vi "Dashboard Main.vi"() -> ()   [LabVIEW 2020]
uses:
  <vilib>/Utility/miscctls.llb/LVRowAndColumnTypeDef.ctl
  <vilib>/event_ctls.llb/eventvkey.ctl
  <vilib>/Rock Robotics/Network Tables/NT Read Numeric Array.vi
  <vilib>/Rock Robotics/Network Tables/NT Read Boolean.vi
  <vilib>/Rock Robotics/WPI/Dashboard/WPI_DashboardLogging Global.vi
panel:
  in  "Camera Settings Right":T1={"Frame Rate"=30, "Compression"=30, "Size"=1, "DB Camera Config"=FALSE} {"Frame Rate" scale=1.0..30.0; "Compression" scale=100.0..-1.0; "Size" items=["640x480", "320x240", "160x120"]}
  in  "Camera Name Right":string(combo)="No Camera Selection"
  out "Camera Perf":string
  in  "Camera Settings":T1={"Frame Rate"=30, "Compression"=30, "Size"=1, "DB Camera Config"=FALSE} {"Frame Rate" scale=1.0..30.0; "Compression" scale=100.0..-1.0; "Size" items=["640x480", "320x240", "160x120"]}
  in  "TCP":refnum<k5>
  in  "Rec Mode":enum32{"Stop", "Record", "Playback"}(radio)
  out "Robot IP":string
  out "Image Message":string="Timeout in Camera Communications"
  in  "Dashboard Tab":T2(tab)
  in  "Select Auto":string(combo)="Select Autonomous ..."
  out "NT Connection":bool
  out "MotorChart R":cluster{"Numeric":dbl, "Numeric":dbl}(graph)
  out "MotorChart L":cluster{"Numeric":dbl, "Numeric":dbl}(graph)
  out "MotorSliders R":cluster{"MotorSlide1":dbl, "MotorSlide2":dbl} {"MotorSlide2" scale=-1.0..1.0 scale format="%#_2e"; "MotorSlide1" scale=-1.0..1.0 scale format="%#_2e"}
  out "MotorSliders L":cluster{"MotorSlide1":dbl, "MotorSlide2":dbl} {"MotorSlide2" scale=-1.0..1.0 scale format="%#_2e"; "MotorSlide1" scale=-1.0..1.0 scale format="%#_2e"}
  out "Gyro":dbl(knob) scale=0.0..360.0
  out "JS1 Z":dbl(slide) scale=-1.0..1.0 scale format="%#_2e"
  out "JS1 Graph":cluster{"X":dbl, "Y":dbl}[](graph)
  out "JS1 Buttons":T3
  out "JS2 Z":dbl(slide) scale=-1.0..1.0 scale format="%#_2e"
  out "JS2 Graph":cluster{"X":dbl, "Y":dbl}[](graph)
  out "JS2 Buttons":T3
  out "Mode":T4(ring)=enum."Auto Disabled"
  out "Right Camera Perf":cluster{"Bandwidth (Mbps)":dbl, "FPS":dbl}
  out "Camera Image Right":T5(plugin-control)
  in  "DB/String 9":string
  in  "DB/String 8":string
  in  "DB/String 7":string
  in  "DB/String 6":string
  in  "DB/String 5":string
  in  "DB/String 4":string
  in  "DB/String 3":string
  in  "DB/String 2":string
  in  "DB/String 1":string
  in  "DB/String 0":string
  in  "DB/Slider 0":dbl(slide) scale=0.0..5.0
  in  "DB/Slider 1":dbl(slide) scale=0.0..5.0
  in  "DB/Slider 2":dbl(slide) scale=0.0..5.0
  in  "DB/Slider 3":dbl(slide) scale=0.0..5.0
  out "DB/LED 3":bool
  out "DB/LED 2":bool
  out "DB/LED 1":bool
  out "DB/LED 0":bool
  in  "DB/Button 3":bool
  in  "DB/Button 2":bool
  in  "DB/Button 1":bool
  in  "DB/Button 0":bool caption="New Name"
  out "Intake on?":bool
  out "Intake Sensor":bool
  out "Elevate Sensor":bool
  in  "Select Climb":string(combo)="Select Autonomous ..."
  in  "Alliance":bool
  in  "Bottom":u32(colorbox)
  out "Last":u32(colorbox)
  out "Intake % Voltage":dbl
  out "Shooter % Voltage":dbl
  in  "Shoot Equation C Value":dbl=3100.0
  in  "Test Slider":dbl(slide) scale=0.0..100.0 scale format="%#_3g"
  in  "On/Off":bool caption="Solenoid"
  in  "Test Name":u16(ring) items=["Select the test to run..."]
  in  "Test Tree":string(tree)
  in  "Motor":cluster{"Value":dbl, "Enable":bool} {"Value" scale=-1.0..1.0 scale format="%#_3g"}
  out "Progress":T6 {"Test Progress" scale=0.0..100.0}
  in  "Rev/Fwd":cluster{"Forward":bool, "Reverse":bool}
  in  "Test Ring":u16(ring) items=["Monochrome", "Color"]
  out "Cmd Status":string
  in  "Execute Command":bool
  in  "Command Params":string[][](table)
  in  "Command Selection":i32(listbox)
  in  "CheckList":i32(listbox)
  out "Tree":string(tree)
  out "Camera Image":T5(plugin-control)
  out "Background":bool
  in  "Camera Name":string(combo)="No Camera Selection"
  # "HW"
  # "HW"
  # "Joysticks"
  # "Drive Motors"
  # "Front"
  # "Right"
  # "Left"
  # "Back"
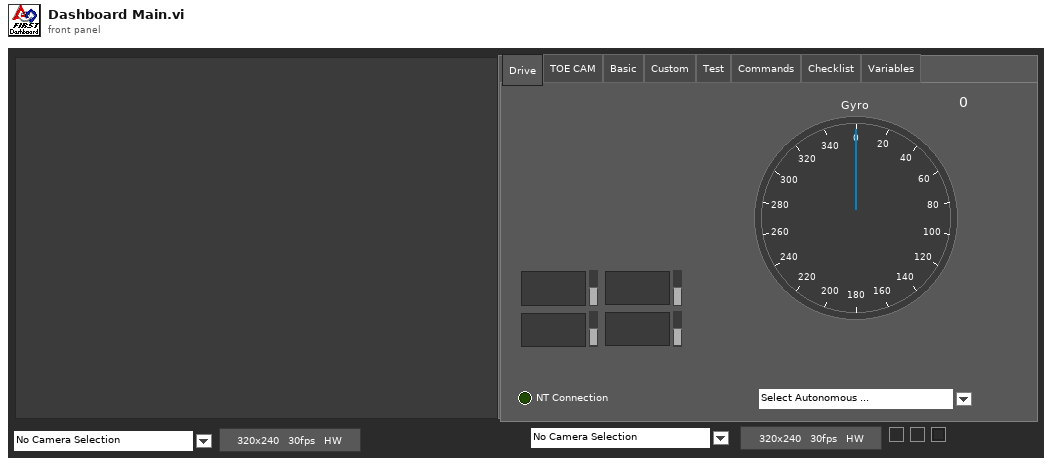
[diagram p1: front panel]
types:
  T1 = cluster{"Frame Rate":i32, "Compression":i32, "Size":u16, "DB Camera Config":bool}
  T2 = enum32{"Drive", "TOE CAM", "Basic", "Custom", "Test", "Commands", "Checklist", "Variables"}
  T3 = cluster{bool, bool, bool, bool, bool, bool, bool, bool, bool, bool, bool, bool}
  T4 = enum8{"Tele-Op Disabled", "Tele-Op Enabled", "Auto Disabled", "Auto Enabled", "Test Disabled", "Test Enabled", "Disconnected", "No Code", "E-Stop"}
  T5 = typedef "IMAQ Image.ctl" = refnum<image>
  T6 = cluster{"Test Progress":u8, "Test Progress Text":string}
  T7 = cluster{"Save Path":path, "Interval (s)":dbl, "Keep":i32}
  T8 = enum32{"Drive", "Camera", "Basic", "Custom", "Test", "Commands", "Checklist", "Variables"}
  T9 = typedef "Image Type" = u32
  T10 = cluster{"IDs":cluster{"RPC field ID":u16, "Unique ID":u16}, "String":string}
  T11 = cluster{"Error Strings":string, "Disable Counts":cluster{u16, u16}, "Rail Faults":cluster{u16, u16, u16}, "Robot IP":string, "DB Mode":u8, "Event Info":cluster{"Name":string, "Type":u8, "Number":u16, "Replay":u8}}
  T12 = cluster{"Storage":cluster{"Disk Free":u64, "RAM Block":u32, "RAM free":u32}, "CPU Utilization":cluster{"CPU % ISR":sgl, "CPU % Time Crit":sgl, "CPU % Timed Str":sgl, "CPU % High":sgl, "CPU % Above":sgl, "CPU % Normal":sgl, "CPU % Low":sgl}, "CAN":cluster{"% Bus Utilization":sgl, "Bus Off Cnt":u32, "TX_FIFO Full Cnt":u32, "Receive Error Cnt":u8, "Transmit Error Cnt":u8}, "HID":cluster{"HID Outputs":u32, "Rumble Low":u16, "Rumble High":u16}[]}
  T13 = cluster{"Status bits":cluster{"Test Mode":bool, "Autonomous":bool, "Enabled":bool, "Code Start":bool, "Brownout":bool, "Reserved 2":bool, "Reserved 3":bool, "E-Stop":bool}, "Code Trace":cluster{"Disabled":bool, "TeleOp":bool, "Auto":bool, "Test":bool}, "Controller Type":enum16{"unknown", "cRIO", "roboRio"}, "Code?":enum16{"unknown", "noCode", "code"}, "Battery V":dbl}
  T14 = cluster{"Control Bits":cluster{"TestMode":bool, "Autonomous":bool, "Enabled":bool, "FMS Present":bool, bool, bool, bool, "E-Stop":bool}, "Team Station ":u8, "Countdown":sgl, "Joystick Values":cluster{"Axes":dbl[], "Buttons":bool[], "POVs":i16[]}[]}
  T15 = cluster{"Axes":dbl[], "Buttons":bool[], "POVs":i16[]}[]
  T16 = cluster{"Axes":dbl[], "Buttons":bool[], "POVs":i16[]}
  T17 = cluster{"Buttons[0]":bool, "Buttons[1]":bool, "Buttons[2]":bool, "Buttons[3]":bool, "Buttons[4]":bool, "Buttons[5]":bool, "Buttons[6]":bool, "Buttons[7]":bool, "Buttons[8]":bool, "Buttons[9]":bool, "Buttons[10]":bool, "Buttons[11]":bool}
  T18 = cluster{"Camera Image":refnum<vi>, "Dashboard Tab":refnum<vi>, "Background":refnum<vi>, "Rec Mode":refnum<vi>, "Test Slider":refnum<vi>, "On/Off ":refnum<vi>, "Test Ring":refnum<vi>, "Rev/Fwd":refnum<vi>, "Test Name":refnum<vi>, "Motor":refnum<vi>, "Progress":refnum<vi>, "CheckList":refnum<vi>, "Tree":refnum<vi>, "Test Tree":refnum<vi>, "Command Params":refnum<vi>, "Command Selection":refnum<vi>, "Execute Command":refnum<vi>, "Cmd Status":refnum<vi>, "Camera Settings":refnum<vi>, "Camera Name":refnum<vi>, "Camera Perf":refnum<vi>, "Camera Settings Right":refnum<vi>, "Camera Name Right":refnum<vi>, "Camera Image Right":refnum<vi>}
  T19 = cluster{"Global Rectangle":i32[], "Contours":cluster{"Contour Type":u32, "ROI Type":u32, "Points":i32[]}[]}
  T20 = cluster{"Camera Name":string, string, "Saved DB Images Info":cluster{"Save Path":path, "Interval (s)":dbl, "Keep":i32}}
  T21 = cluster{"Camera Name Right":string, string, "Saved DB Images Info":cluster{"Save Path":path, "Interval (s)":dbl, "Keep":i32}}
  T22 = cluster{"Operation":enum16{"Update", "Clear"}, "Color Box":u32}[]
  T23 = typedef "eventvkey.ctl" = enum16{"ASCII", "Enter", "Return", "Shift", "Ctrl", "Alt", "Cmd", "Opt", "Caps", "NumLock", "Clear", "Break", "Up", "Down", "Left", "Right", "Insert", "Delete", "Home", "End", "PageUp", "PageDown", "Escape", "Help", "Pause", "ScrollLock", "F1", "F2", "F3", "F4", "F5", "F6", "F7", "F8", "F9", "F10", "F11", "F12", "F13", "F14", "F15", "F16", "F17", "F18", "F19", "F20", "F21", "F22", "F23", "F24", "Play", "VolumeUp", "VolumeDown", "Mute", "Two Byte Char"}
  T24 = cluster{"Image Size":bool, "Image Type":bool, "Pixel Value":bool, "ROI Information":bool, "Zoom Factor":bool}
  T25 = cluster{"Operation":enum16{"Update", "Clear"}, "Color Box":u32}
  T26 = typedef "LVRowAndColumnTypeDef.ctl" = cluster{"Row":i32, "Column":i32}
  T27 = cluster{"Shift":bool, "Ctrl":bool, "Alt":bool, "Cmd":bool, "Opt":bool}
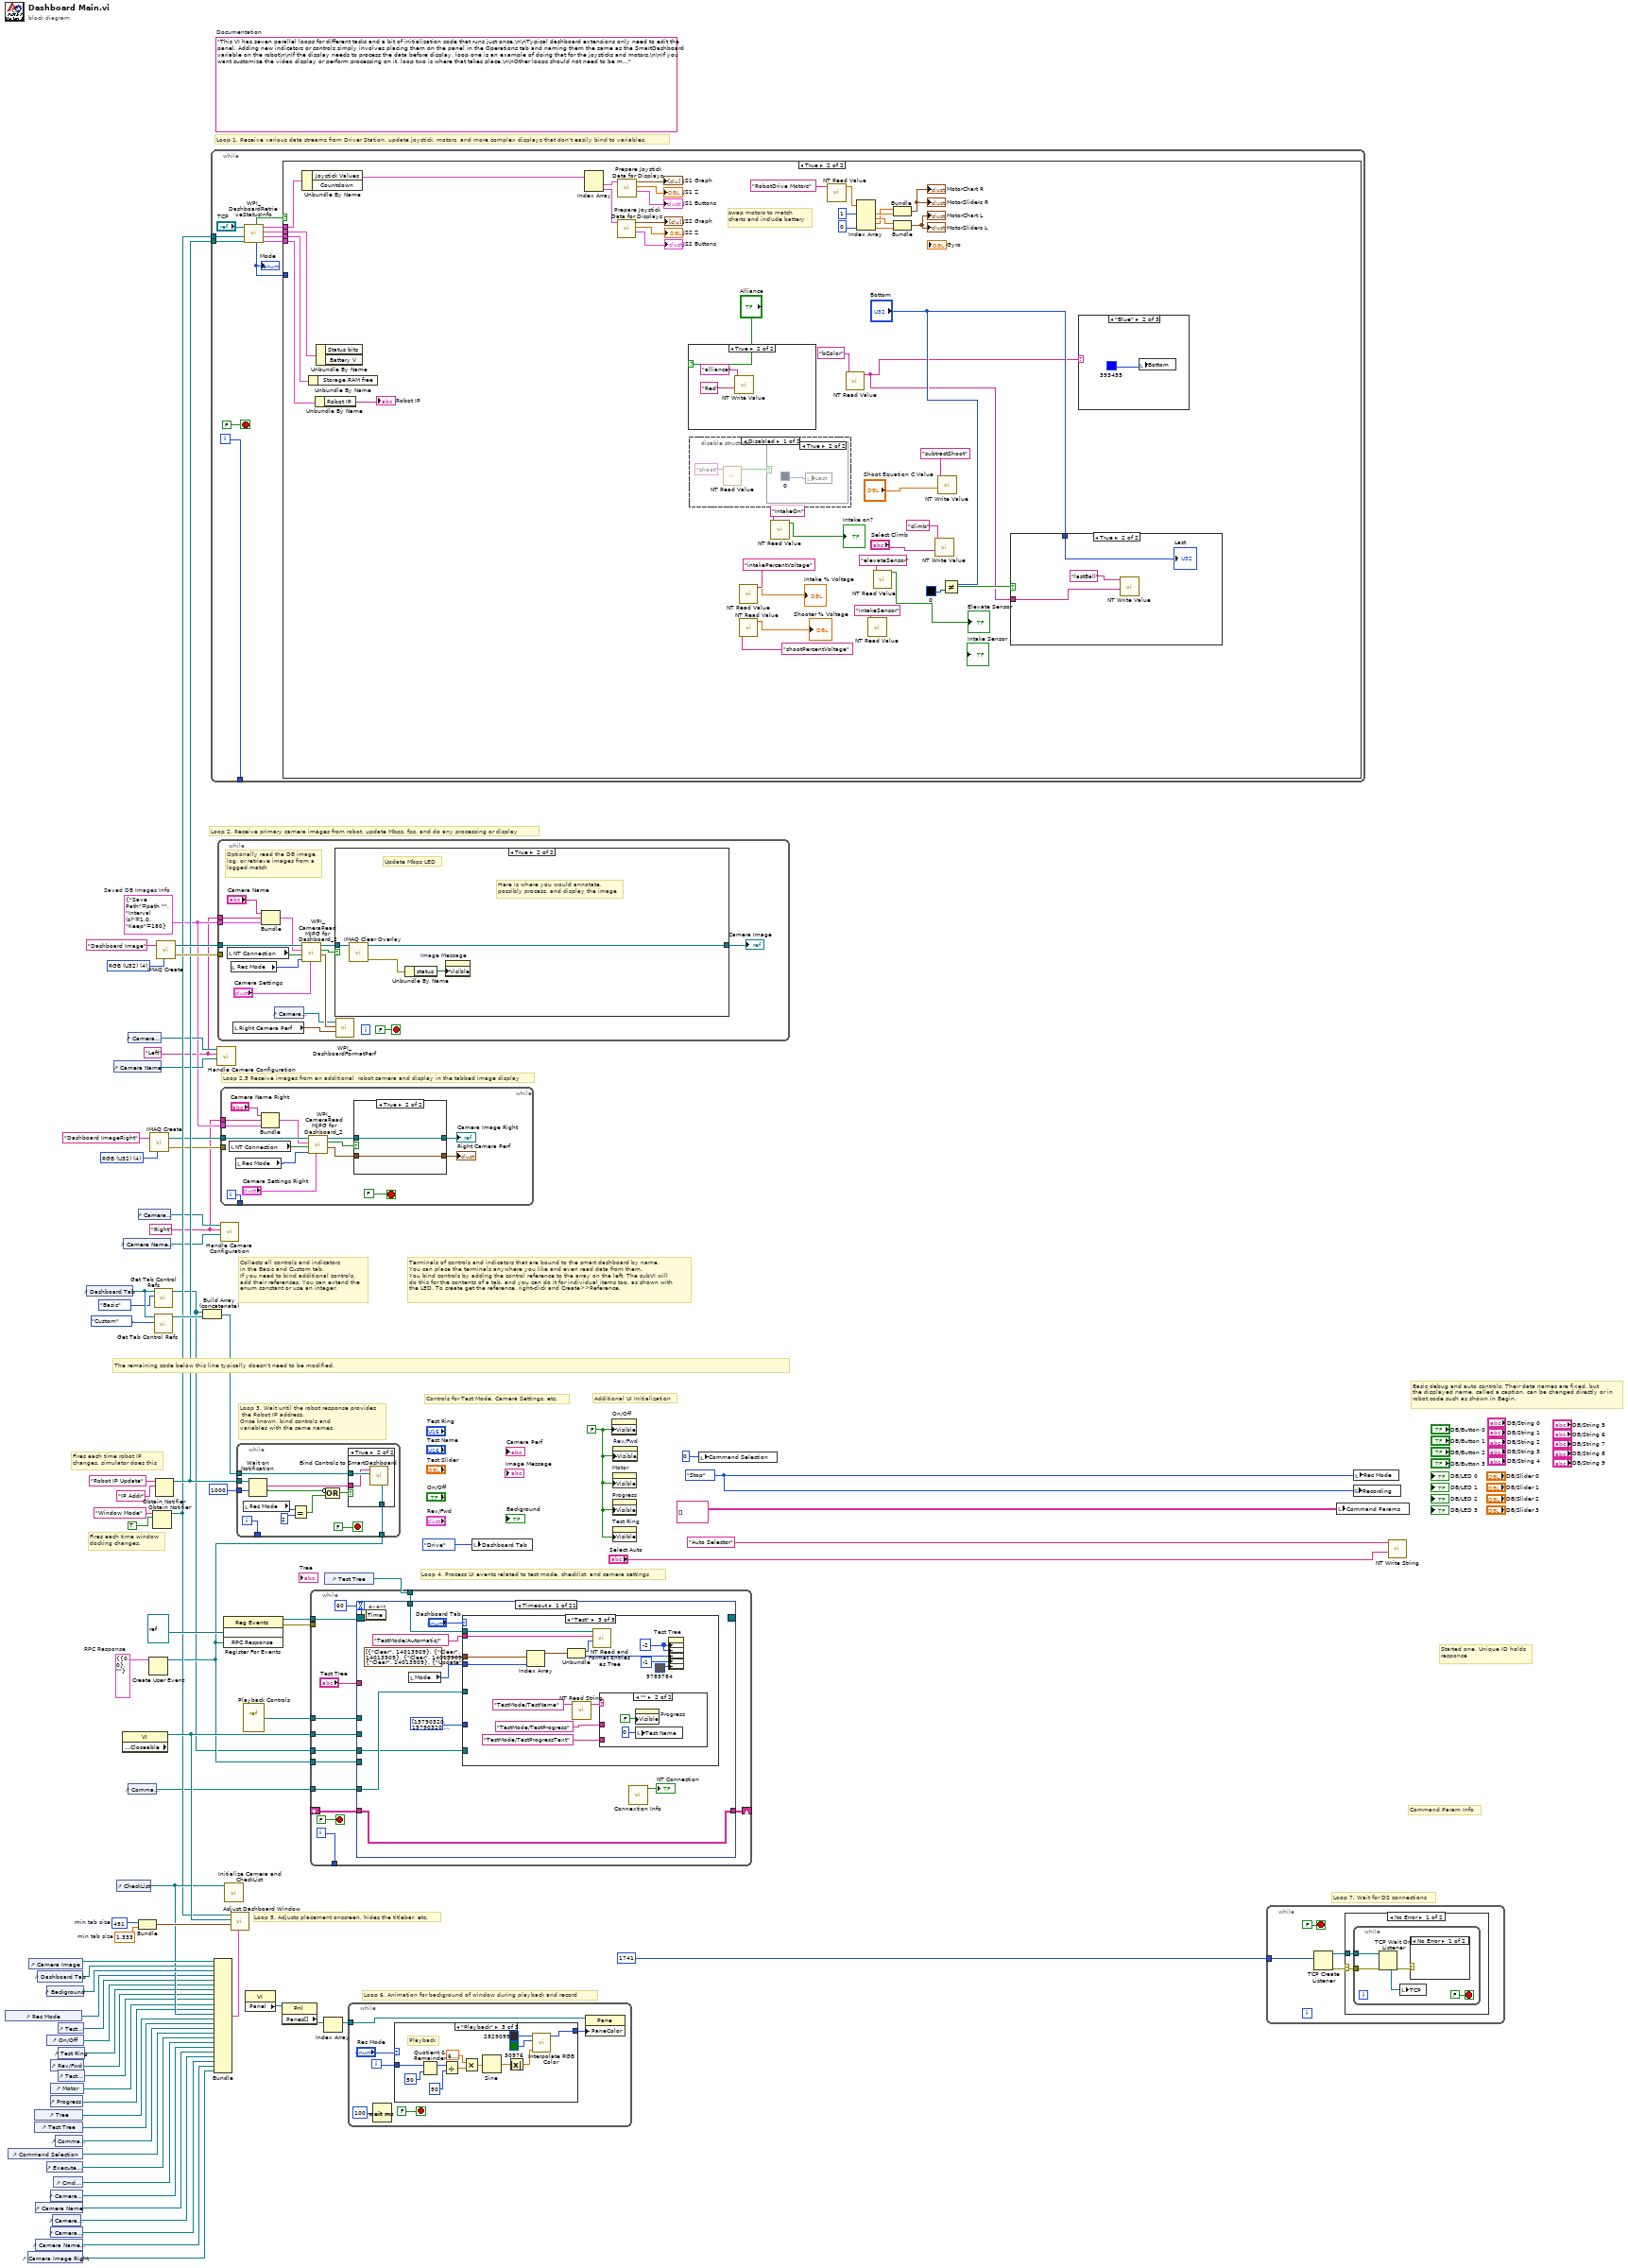
[diagram p0: block diagram]
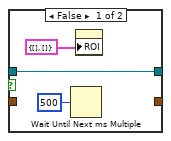
[diagram p2: hidden frame]
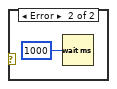
[diagram p3: hidden frame]
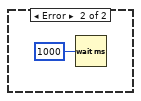
[diagram p4: hidden frame]
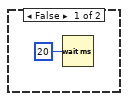
[diagram p5: hidden frame]
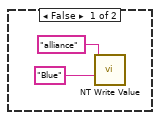
[diagram p9: hidden frame]
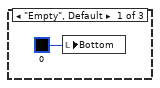
[diagram p10: hidden frame]
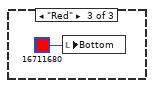
[diagram p11: hidden frame]
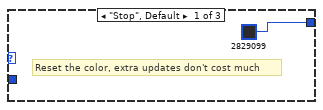
[diagram p12: hidden frame]
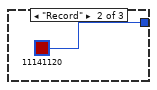
[diagram p13: hidden frame]
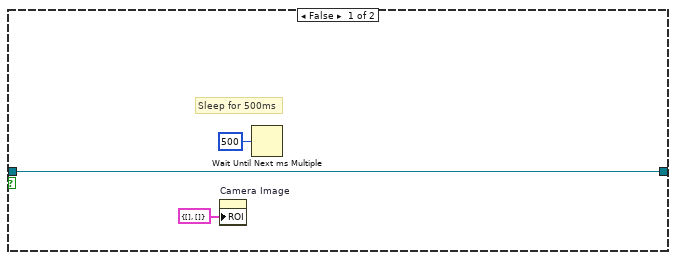
[diagram p15: hidden frame]
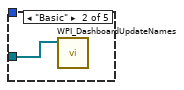
[diagram p17: hidden frame]
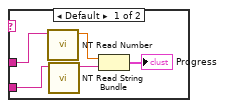
[diagram p18: hidden frame]
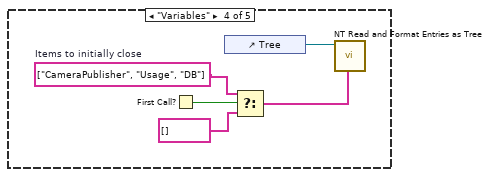
[diagram p19: hidden frame]
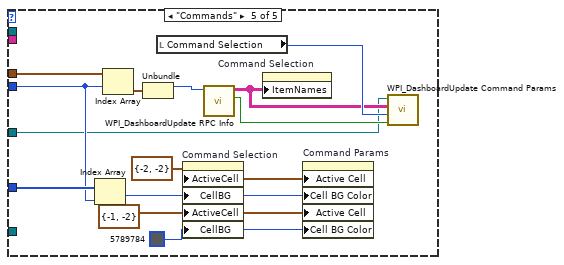
[diagram p20: hidden frame]
diagram:
  w3 = T7 {"Save Path"=path "", "Interval (s)"=1.0, "Keep"=180}  # Saved DB Images Info
  w2 = "Right"
  w1 = "Left"
  w13 = T9 4 items=["Grayscale (U8)", "Grayscale (I16)", "Grayscale (SGL)", "Complex (CSG)", "RGB (U32)", "HSL (U32)", "RGB (U64)"] ("Image Type")
  w29 = T10 {"IDs"={"RPC field ID"=0, "Unique ID"=0}, "String"=""}  # RPC Response
  w52 = 491  # min tab size
  w51 = 1.333  # min tab size
  w59 = enum32{"Stop", "Record", "Playback"}."Stop" ("Rec Mode")
  w36 = FALSE ("Visible")
  (unwired) "This VI has seven parallel loops for different tasks and a bit of initialization code that runs just once.\n\nTypical dashboard extensions only need to edit the panel. Adding new indicators or controls simply involves placing them on the panel in the Operations tab and naming them the same as the SmartDashboard variable on the robot\n\nIf the display needs to process the data before display, loop one is an example of doing that for the joysticks and motors.\n\nIf you want customize the video display or perform processing on it, loop two is where that takes place.\n\nOther loops should not need to be modified. They are pretty standard, and document the task they perform."  # Documentation
  w76 = T9 4 items=["Grayscale (U8)", "Grayscale (I16)", "Grayscale (SGL)", "Complex (CSG)", "RGB (U32)", "HSL (U32)", "RGB (U64)"] ("Image Type")
  # "Loop 2.5 Receive images from an additional  robot camera and display in the tabbed image display"
  # "Command Param Info"
  # "Started one, Unique ID holds\nresponse"
  # "Loop 7. Wait for DS connections"
  # "Basic debug and auto controls: Their data names are fixed, but\nthe displayed name, called a caption, can be changed directly or in\nrobot code such as shown in Begin."
  # "Controls for Test Mode, Camera Settings, etc."
  # "Additional UI Initialization"
  # "Loop 6. Animation for background of window during playback and record"
  # "Fires each time robot IP\nchanges, simulator does this"
  # "Fires each time window\ndocking changes."
  # "Collects all controls and indicators\nin the Basic and Custom tab.\nIf you need to bind additional controls,\nadd their references. You can extend the\nenum constant or use an integer."
  # "The remaining code below this line typically doesn't need to be modified."
  # "Loop 4. Process UI events related to test mode, checklist, and camera settings"
  # "Terminals of controls and indicators that are bound to the smart dashboard by name.\nYou can place the terminals anywhere you like and even read data from them.\nYou bind controls by adding the control reference to the array on the left. The subVI will\ndo this for the contents of a tab, and you can do it for individual items too, as shown with\nthe LED. To create get the reference, right-click and Create>>Reference."
  # "Loop 3. Wait until the robot response provides\n the Robot IP address.\nOnce known, bind controls and\nvariables with the same names."
  # "Loop 5. Adjusts placement onscreen, hides the titlebar, etc."
  # "Loop 1. Receive various data streams from Driver Station, update joystick, motors, and more complex displays that don't easily bind to variables."
  # "Loop 2. Receive primary camera images from robot, update Mbps, fps, and do any processing or display"
  n1 = control-ref of="Rec Mode"() -> (w42:refnum<vi>)
  n2 = control-ref of="Command Selection"() -> (w28:refnum<vi>)
  n3 = control-ref of="Camera Image Right"() -> (w6:refnum<vi>)
  n4 = control-ref of="Camera Image"() -> (w54:refnum<vi>)
  n5 = control-ref of="Tree"() -> (w46:refnum<vi>)
  n6 = control-ref of="Test Tree"() -> (w45:refnum<vi>)
  n7 = control-ref of="Camera Name"() -> (w19:refnum<vi>)
  n8 = control-ref of="Camera Name Right"() -> (w7:refnum<vi>)
  n9 = control-ref of="Dashboard Tab"() -> (w53:refnum<vi>)
  n10 = control-ref of="Execute Command"() -> (w30:refnum<vi>)
  n11 = control-ref of="Background"() -> (w49:refnum<vi>)
  n12 = control-ref of="On/Off"() -> (w40:refnum<vi>)
  n13 = control-ref of="Progress"() -> (w37:refnum<vi>)
  n14 = control-ref of="Camera Settings"() -> (w20:refnum<vi>)
  n15 = control-ref of="Camera Settings Right"() -> (w8:refnum<vi>)
  n16 = control-ref of="Rev/Fwd"() -> (w38:refnum<vi>)
  n17 = control-ref of="Motor"() -> (w43:refnum<vi>)
  n18 = control-ref of="Camera Perf"() -> (w18:refnum<vi>)
  n19 = control-ref of="Cmd Status"() -> (w24:refnum<vi>)
  n20 = control-ref of="Command Params"() -> (w31:refnum<vi>)
  n21 = control-ref of="Test Slider"() -> (w41:refnum<vi>)
  n22 = control-ref of="Test Ring"() -> (w39:refnum<vi>)
  n23 = control-ref of="Test Name"() -> (w44:refnum<vi>)
  n24 = control-ref of="Dashboard Tab"() -> (w57:refnum<vi>)
  n25 = control-ref of="Camera Name"() -> (w21:refnum<vi>)
  n26 = control-ref of="CheckList"() -> (w47:refnum<vi>)
  n27 = property class="VI" props=["Front Panel.Closeable"]() -> (reference out=w58:refnum<vi>)  [unwired: 2 in, 2 out]
  n28 = control-ref of="Camera Name Right"() -> (w9:refnum<vi>)
  n29 = control-ref of="Camera Settings"() -> (w22:refnum<vi>)
  n30 = control-ref of="Command Params"() -> (w23:refnum<vi>)
  n31 = control-ref of="Camera Settings Right"() -> (w10:refnum<vi>)
  n32 = Bundle("min tab size"=w52, "min tab size"=w51) -> (w50:cluster{"min tab size":i32, "min tab size":dbl})  [unwired: 1 in]
  n33 = Create User Event(user event datatype=w29) -> (user event=w25:refnum<user-event>)  [unwired: 1 in, 1 out]
  n34 = call "IMAQ Create"("Image Name"="Dashboard ImageRight", "Image Type"=w13) -> ("New Image"=w12:T5, "error out"=w11:errorcluster)  [unwired: 2 in, 1 out]
  n35 = Obtain Notifier(name (unnamed)="Window Mode", notification data type=TRUE) -> (notifier out=w34:refnum<notifier>)  [unwired: 2 in, 2 out]
  n36 = call <vilib>:"Get Tab Control Refs.vi"("Page Index"=T8."Basic" ("Dashboard Tab"), "TabControl in"=w57) -> ("ControlsOnPage"=w17:refnum<vi>[])  [unwired: 9 in]
  n37 = call <vilib>:"Get Tab Control Refs.vi"("Page Index"=T8."Custom" ("Dashboard Tab"), "TabControl in"=w57) -> ("ControlsOnPage"=w56:refnum<vi>[])  [unwired: 9 in]
  n38 = Obtain Notifier(name (unnamed)="Robot IP Update", notification data type="IP Addr" ("name (unnamed)")) -> (notifier out=w35:refnum<notifier>)  [unwired: 2 in, 2 out]
  n39 = call "IMAQ Create"("Image Name"="Dashboard Image", "Image Type"=w76) -> ("New Image"=w74:T5, "error out"=w73:errorcluster)  [unwired: 2 in, 1 out]
  n40 = Build Array (concatenate)(w17, w56) -> (w55:refnum<vi>[])
  n41 = while {
    tunnel: [w86] -> _
    tunnel: w35 -> [w80]
    tunnel: w34 -> [w77]
    i -> [w86]
    stop <- FALSE stop-if-true
    n42 = call <vilib>:"WPI_DashboardRetrieveStatusInfo.vi"("Binding Refnum"=w80, "Window Mode Notifier"=w77, "TCP Cnx"="TCP") -> ("Power and Errors"=w81:T11, "Robot Metrics"=w84:T12, "Status Info"=w85:T13, "Control Info"=w82:T14, "Robot Mode"=w79:T4, "Process?"=w83:bool)  [unwired: 3 in]
    "Mode" <- w79
    n43 = case shown="True" w83 {
      tunnel: w85 -> [_ w131]
      tunnel: w84 -> [_ w130]
      tunnel: w82 -> [_ w129]
      tunnel: w81 -> [_ w128]
      tunnel: w79 -> [_ _]
      frame False {
        n44 = Wait (ms)(milliseconds to wait=u32 20) -> ()  [unwired: 1 out]
      }
      frame True {
        # "swap motors to match\ncharts and include battery"
        n45 = Unbundle By Name(w129) -> ("Joystick Values"=w119:T15)  [unwired: 1 out]
        n46 = Unbundle By Name(w130) -> ()  [unwired: 1 out]
        n47 = Unbundle By Name(w128) -> ("Robot IP"=→"Robot IP":string)
        n48 = Unbundle By Name(w131) -> ()  [unwired: 2 out]
        n49 = Index Array(array=w119) -> (element #1=w118:T16, element #2=w114:T16)  [unwired: 2 in]
        n50 = call "Prepare Joystick Data for Displays.vi"("Joystick Values"=w114) -> ("Buttons"=→"JS2 Buttons":T17, "Z Axis"=→"JS2 Z":dbl, "Cartesian Data"=→"JS2 Graph":cluster{"X axis":dbl, "X axis":dbl}[])  [unwired: 8 in]
        n51 = call "Prepare Joystick Data for Displays.vi"("Joystick Values"=w118) -> ("Buttons"=→"JS1 Buttons":T17, "Z Axis"=→"JS1 Z":dbl, "Cartesian Data"=→"JS1 Graph":cluster{"X axis":dbl, "X axis":dbl}[])  [unwired: 8 in]
        n52 = case shown="True" "Alliance" {
          frame False {
            n53 = call-poly <vilib>:"NT Write Value.vi"("String"="Blue", "Name"="alliance") -> ()  [unwired: 9 in, 1 out]
          }
          frame True {
            n54 = call-poly <vilib>:"NT Write Value.vi"("String"="Red", "Name"="alliance") -> ()  [unwired: 9 in, 1 out]
          }
        }
        n55 = disable-structure shown="Disabled" {
          frame Disabled {
            n56 = call-poly <vilib>:"NT Read Value.vi"("Name"="shoot") -> ("Boolean"=w136:bool)  [unwired: 9 in, 1 out]
            n57 = case shown="True" w136 {
              frame False {
              }
              frame True {
                n58 = local write "Last"(u32 0 ("Top")) -> ()
              }
            }
          }
          frame Enabled {
          }
        }
        n59 = call-poly <vilib>:"NT Read Value.vi"("Name"="intakePercentVoltage") -> ("Numeric"=→"Intake % Voltage":dbl)  [unwired: 9 in, 1 out]
        n60 = call-poly <vilib>:"NT Read Value.vi"("Name"="shootPercentVoltage") -> ("Numeric"=→"Shooter % Voltage":dbl)  [unwired: 9 in, 1 out]
        n61 = call-poly <vilib>:"NT Read Value.vi"("Name"="IntakeOn") -> ("Boolean"=→"Intake on?":bool)  [unwired: 9 in, 1 out]
        n62 = call-poly <vilib>:"NT Read Value.vi"("Name"="RobotDrive Motors") -> ("Numeric Array"=w109:dbl[])  [unwired: 9 in, 1 out]
        n63 = call-poly <vilib>:"NT Read Value.vi"("Name"="bColor") -> ("String"=w102:string)  [unwired: 9 in, 1 out]
        n64 = Index Array(array=w109, index #1=1, index #4=0) -> (element #1=w123:dbl, element #2=w124:dbl, element #3=w122:dbl, element #4=w127:dbl)  [unwired: 2 in]
        n65 = call-poly <vilib>:"NT Read Value.vi"("Name"="intakeSensor") -> ()  [unwired: 9 in, 2 out]
        n66 = call-poly <vilib>:"NT Read Value.vi"("Name"="elevateSensor") -> ("Boolean"=→"Elevate Sensor":bool)  [unwired: 9 in, 1 out]
        n67 = Bundle("Numeric"=w122, "Numeric"=w123) -> (→"MotorChart R" →"MotorSliders R":cluster{"Numeric":dbl, "Numeric":dbl})  [unwired: 1 in]
        n68 = Bundle("Numeric"=w124, "Numeric"=w127) -> (→"MotorChart L" →"MotorSliders L":cluster{"Numeric":dbl, "Numeric":dbl})  [unwired: 1 in]
        n69 = call-poly <vilib>:"NT Write Value.vi"("String"="Select Climb", "Name"="climb") -> ()  [unwired: 9 in, 1 out]
        n70 = call-poly <vilib>:"NT Write Value.vi"("Numeric"="Shoot Equation C Value", "Name"="subtractShoot") -> ()  [unwired: 9 in, 1 out]
        n71 = Not Equal?(x="Bottom", y=u32 0 ("Bottom")) -> (x != y?=w105:bool)
        n72 = case shown="True" w105 {
          tunnel: "Bottom" -> [_ w133]
          tunnel: w102 -> [_ w132]
          frame False {
          }
          frame True {
            n73 = call-poly <vilib>:"NT Write Value.vi"("String"=w132, "Name"="lastBall") -> ()  [unwired: 9 in, 1 out]
            "Last" <- w133
          }
        }
        n74 = case shown="\"Blue\"" w102 {
          frame "Empty", Default {
            n75 = local write "Bottom"(u32 0 ("Bottom")) -> ()
          }
          frame "Blue" {
            n76 = local write "Bottom"(u32 393455 ("Turret")) -> ()
          }
          frame "Red" {
            n77 = local write "Bottom"(u32 16711680 ("Bottom")) -> ()
          }
        }
      }
    }
  }
  n78 = Bundle("Camera Image"=w54, "Dashboard Tab"=w53, "Background"=w49, "Rec Mode"=w42, "Test Slider"=w41, "On/Off"=w40, "Test Ring"=w39, "Rev/Fwd"=w38, "Test Name"=w44, "Motor"=w43, "Progress"=w37, "CheckList"=w47, "Tree"=w46, "Test Tree"=w45, "Command Params"=w31, "Command Selection"=w28, "Execute Command"=w30, "Cmd Status"=w24, "Camera Settings"=w20, "Camera Name"=w19, "Camera Perf"=w18, "Camera Settings Right"=w8, "Camera Name Right"=w7, "Camera Image Right"=w6) -> (w48:T18)  [unwired: 1 in]
  n79 = call "Handle Camera Configuration.vi"("CameraNameRef"=w21, "Display Name"=w1, "ClusterRef"=w22) -> ()  [unwired: 9 in]
  n80 = while {
    tunnel: w74 -> [w158]
    tunnel: w73 -> [_]
    tunnel: w3 -> [w151]
    tunnel: w1 -> [w148]
    stop <- FALSE stop-if-true
    # "Optionally read the DB image,\nlog, or retrieve images from a\nlogged match"
    n81 = local read "NT Connection"() -> (w152:bool)
    n82 = local read "Rec Mode"() -> (w155:enum32{"Stop", "Record", "Playback"})
    n83 = local read "Right Camera Perf"() -> (w146:cluster{"Bandwidth (Mbps)":dbl, "FPS":dbl})
    n84 = Bundle("Camera Name"="Camera Name", w148, "Saved DB Images Info"=w151) -> (w150:T20)  [unwired: 1 in]
    n85 = control-ref of="Camera Perf"() -> (w145:refnum<vi>)
    n86 = call <vilib>:"WPI_CameraRead MJPG for Dashboard_2.vi"("Camera Settings"="Camera Settings", "Rec Mode"=w155, "NT Connection"=w152, "Capture Info"=w150, "Image in"=w158) -> ("perf info"=w147:cluster{"Bandwidth (Mbps)":dbl, "fps":dbl}, "Active"=w156:bool, "Image\\ out"=w157:T5)  [unwired: 4 in]
    n87 = case shown="True" w156 {
      tunnel: w157 -> [w161 w164]
      tunnel: [w161 w163] -> w153
      frame False {
        # "Sleep for 500ms"
        n88 = property on="Camera Image" class="ImageControl"("ROI"=T19 {"Global Rectangle"=[], "Contours"=[]}) -> ()  [unwired: 2 in, 2 out]
        n89 = Wait Until Next ms Multiple(millisecond multiple=u32 500) -> ()  [unwired: 1 out]
      }
      frame True {
        # "Here is where you would annotate,\npossibly process, and display the image"
        # "Update Mbps LED"
        n90 = call "IMAQ Clear Overlay"("Image"=w164) -> ("error out"=w165:errorcluster, "Image Out"=w163:T5)  [unwired: 2 in, 7 out]
        n91 = Unbundle By Name(w165) -> ("status"=w166:bool)
        n92 = property on="Image Message" class="Str"("Visible"=w166) -> ()  [unwired: 2 in, 2 out]
      }
    }
    "Camera Image" <- w153
    n93 = call <vilib>:"WPI_DashboardFormatPerf.vi"("Right Camera Perf"=w146, "Performance"=w147, "String in"=w145) -> ()  [unwired: 9 in]
  }
  n94 = call "Handle Camera Configuration.vi"("CameraNameRef"=w9, "Display Name"=w2, "ClusterRef"=w10) -> ()  [unwired: 9 in]
  n95 = while {
    tunnel: w12 -> [w181]
    tunnel: w11 -> [_]
    tunnel: [w176] -> _
    tunnel: w3 -> [w172]
    tunnel: w2 -> [w169]
    i -> [w176]
    stop <- FALSE stop-if-true
    n96 = local read "NT Connection"() -> (w173:bool)
    n97 = local read "Rec Mode"() -> (w180:enum32{"Stop", "Record", "Playback"})
    n98 = Bundle("Camera Name Right"="Camera Name Right", w169, "Saved DB Images Info"=w172) -> (w171:T21)  [unwired: 1 in]
    n99 = call <vilib>:"WPI_CameraRead MJPG for Dashboard_2.vi"("Camera Settings"="Camera Settings Right", "Rec Mode"=w180, "NT Connection"=w173, "Capture Info"=w171, "Image in"=w181) -> ("perf info"=w167:cluster{"Bandwidth (Mbps)":dbl, "fps":dbl}, "Active"=w175:bool, "Image\\ out"=w178:T5)  [unwired: 4 in]
    n100 = case shown="True" w175 {
      tunnel: w178 -> [w183 w186]
      tunnel: [w183 w186] -> w174
      tunnel: [_ w185] -> w168
      tunnel: w167 -> [_ w185]
      frame False {
        n101 = Wait Until Next ms Multiple(millisecond multiple=u32 500) -> ()  [unwired: 1 out]
        n102 = property on="Camera Image Right" class="ImageControl"("ROI"=T19 {"Global Rectangle"=[], "Contours"=[]}) -> ()  [unwired: 2 in, 2 out]
      }
      frame True {
      }
    }
    "Camera Image Right" <- w174
    "Right Camera Perf" <- w168
  }
  n103 = register-events(refnum<vi> refnum, w25) -> (reference out=w63:refnum<event-registration>, error out=w62:errorcluster)  [unwired: 2 in]
  n104 = call "Initialize Camera and CheckList.vi"("ListBox in"=w47) -> ()  [unwired: 11 in]
  n105 = call "Adjust Dashboard Window.vi"("Sizing Refnums"=w48, "Size Constraints"=w50, "VI"=w58, "WIn Mode"=w34) -> ()  [unwired: 8 in]
  n106 = while {
    tunnel: w55 -> [w198]
    tunnel: w35 -> [w196]
    tunnel: [w194] -> _
    tunnel: u32 1000 ("milliseconds to wait") -> [w193]
    tunnel: w25 -> [w187]
    i -> [w194]
    stop <- FALSE stop-if-true
    n107 = local read "Rec Mode"() -> (w189:enum32{"Stop", "Record", "Playback"})
    n108 = Wait on Notification(notifier=w196, timeout in ms (-1)=w193) -> (notification=w195:string, timed out?=w191:bool)  [unwired: 2 in, 2 out]
    n109 = Equal?(x=w189, y=u16 2 ("Rec Mode")) -> (x = y?=w190:bool)
    n110 = Compound Arithmetic op=OR(invert w191, w190) -> (w192:bool)
    n111 = case shown="True" w192 {
      tunnel: w198 -> [_ w201]
      tunnel: w195 -> [_ w200]
      tunnel: w187 -> [_ w199]
      frame False {
      }
      frame True {
        n112 = call <vilib>:"Bind Controls to SmartDashboard.vi"("RPC ref"=w199, "Bound Control Refs"=w201, "Server IP Address"=w200) -> ()  [unwired: 9 in]
      }
    }
  }
  n113 = vi-ref "Playback Controls.vi"() -> (w64:refnum<vi>)
  n114 = property class="VI"() -> ("Panel"=w66:refnum<vi>)  [unwired: 2 in, 2 out]
  n115 = property class="Pnl"(reference=w66) -> ("Panes[]"=w67:refnum<vi>[])  [unwired: 1 in, 2 out]
  n116 = Index Array(array=w67) -> (element=w65:refnum<vi>)  [unwired: 1 in]
  n117 = control-ref of="Test Tree"() -> (w68:refnum<vi>)
  n118 = while {
    tunnel: [w211] -> _
    tunnel: w68 -> [w210]
    tunnel: w64 -> [w209]
    tunnel: w63 -> [w208]
    tunnel: w62 -> [_]
    tunnel: w58 -> [w207]
    tunnel: w25 -> [w206]
    tunnel: w23 -> [w205]
    shift-right: [w204] -> _
    shift-left: _ -> [w203]
    tunnel: w17 -> [w202]
    i -> [w211]
    stop <- FALSE stop-if-true
    n119 = event shown="[0] Timeout" {
      selector: w208 -> [_ _ _ _ _ _ _ _ _ _ _ _ _ _ _ _ _ _ _ _ _]
      dyn-events: [_ _ _ _ _ _ _ _ _ _ _ _ _ _ _ _ w471 _ _ _ _] -> _
      timeout: u32 60 ("milliseconds to wait") -> [_ _ _ _ _ _ _ _ _ _ _ _ _ _ _ _ _ _ _ _ _]
      tunnel: w210 -> [w223 _ _ _ _ _ _ _ _ _ _ _ _ _ _ _ _ _ _ _ _]
      tunnel: "Test Tree" -> [_ _ _ _ _ _ _ _ _ _ _ w438 w446 w448 w452 w460 _ _ _ _ _]
      tunnel: w209 -> [_ _ _ _ _ _ _ _ _ _ _ _ _ _ _ _ w473 _ w491 _ _]
      tunnel: w207 -> [_ _ _ _ _ _ _ _ _ _ _ _ _ _ _ _ w469 _ _ _ _]
      tunnel: w206 -> [_ _ _ _ _ _ _ _ _ _ _ _ _ _ _ _ w467 _ _ _ _]
      tunnel: w205 -> [w218 _ _ _ _ _ w389 _ _ _ _ _ _ _ _ _ _ _ _ _ _]
      tunnel: [w217 w266 w368 w373 w382 w386 w387 w396 w406 w413 w425 w437 w444 w447 w451 w459 w466 w486 w488 w492 w505] -> w204
      tunnel: w203 -> [w217 w266 w368 w373 w382 w386 w387 _ _ w413 w425 w437 w444 w447 w451 w459 w466 w486 w488 w492 w505]
      tunnel: w202 -> [w215 _ _ _ _ _ _ _ _ _ _ _ _ _ _ _ _ _ _ _ _]
      event Timeout {
        n120 = event-data() -> ()  [unwired: 1 in, 1 out]
        n121 = local read "Mode"() -> (w220:T4)
        n122 = case shown="\"Test\"" "Dashboard Tab" {
          tunnel: w223 -> [_ _ w239 _ _]
          tunnel: "TestMode/Automatic/" ("Name Pattern") -> [_ _ w238 _ _]
          tunnel: T22 [{"Operation"=enum."Clear", "Color Box"=14013909}, {"Operation"=enum."Clear", "Color Box"=14013909}, {"Operation"=enum."Clear", "Color Box"=14013909}, {"Operation"=enum."Clear", "Color Box"=14013909}, {"Operation"=enum."Update", "Color Box"=14013909}, {"Operation"=enum."Update", "Color Box"=16777215}, {"Operation"=enum."Clear", "Color Box"=14013909}, {"Operation"=enum."Clear", "Color Box"=14013909}, {"Operation"=enum."Clear", "Color Box"=14013909}] -> [_ _ w231 _ w259]
          tunnel: w220 -> [_ _ w230 _ w258]
          tunnel: u32[] [15790320, 15790320, 15790320, 15790320, 16777215, 16777215, 15790320, 15790320, 15790320] -> [_ _ _ _ w264]
          tunnel: w218 -> [_ _ _ _ w252]
          tunnel: w215 -> [_ w225 _ _ _]
          frame "Custom", Default {
          }
          frame "Basic" {
            n123 = call <vilib>:"WPI_DashboardUpdateNames.vi"("Controls on Tab"=w225) -> ()  [unwired: 11 in]
          }
          frame "Test" {
            w237 = -2 ("Active Item:Row Number")
            n124 = Index Array(array=w231, index=w230) -> (element=w232:T25)
            n125 = Unbundle(w232) -> ("Operation"=w233:enum16{"Update", "Clear"}, "Color Box"=w234:u32)
            n126 = call <vilib>:"NT Read String.vi"("Name"="TestMode/TestName") -> ("String"=w228:string)  [unwired: 9 in, 1 out]
            n127 = call <vilib>:"NT Read and Format Entries as Tree.vi"("Operation"=w233, "Name Pattern"=w238, "Tree Refnum"=w239) -> ()  [unwired: 7 in, 2 out]
            n128 = case shown="\"\"" w228 {
              tunnel: "TestMode/TestProgress" ("Name") -> [w241 _]
              tunnel: "TestMode/TestProgressText" ("Name") -> [w240 _]
              frame Default {
                n129 = call <vilib>:"NT Read Number.vi"("Name"=w241) -> ("Numeric"=w242:dbl)  [unwired: 9 in, 1 out]
                n130 = call <vilib>:"NT Read String.vi"("Name"=w240) -> ("String"=w243:string)  [unwired: 9 in, 1 out]
                n131 = Bundle("Numeric"=w242, "String"=w243) -> (→"Progress":cluster{"Numeric":dbl, "String":string})  [unwired: 1 in]
              }
              frame "" {
                n132 = property on="Progress" class="Clust (strict)"("Visible"=FALSE) -> ()  [unwired: 2 in, 2 out]
                n133 = local write "Test Name"(u16 0) -> ()
              }
            }
            n134 = property on="Test Tree" class="Tree (strict)"("Active Item Row Number"=w237, "ActiveColNum"=w237, "CellBG"=w234, "Active Item Row Number"=-1 ("Active Item:Row Number"), "CellBG"=u32 5789784 ("Color Box")) -> ()  [unwired: 2 in, 2 out]
          }
          frame "Variables" {
            w249 = string[] ["CameraPublisher", "Usage", "DB"]  # Items to initially close
            n135 = First Call?() -> (First Call?: T/F=w250:bool)
            n136 = control-ref of="Tree"() -> (w251:refnum<vi>)
            n137 = Select(t=w249, s=w250, f=string[] []) -> (s? t:f=w247:string[])
            n138 = call <vilib>:"NT Read and Format Entries as Tree.vi"("Tags to  Close"=w247, "Tree Refnum"=w251) -> ()  [unwired: 8 in, 2 out]
          }
          frame "Commands" {
            w260 = u32 5789784 ("Color Box")
            w261 = T26 {"Row"=-1, "Column"=-2} ("Active Cell:Active Cell")
            w263 = T26 {"Row"=-2, "Column"=-2} ("Active Cell:Active Cell")
            n139 = Index Array(array=w264, index=w258) -> (element=w262:u32)
            n140 = Index Array(array=w259, index=w258) -> (element=w257:T25)
            n141 = Unbundle(w257) -> ("Operation"=w256:enum16{"Update", "Clear"})  [unwired: 1 out]
            n142 = local read "Command Selection"() -> (w255:i32)
            n143 = property on="Command Selection" class="MCListbox (strict)"("ActiveCell"=w263, "CellBG"=w262, "ActiveCell"=w261, "CellBG"=w260) -> ()  [unwired: 2 in, 2 out]
            n144 = call <vilib>:"WPI_DashboardUpdate RPC Info.vi"("Operation"=w256) -> ("update"=w254:bool, "commands"=w253:string[][])  [unwired: 9 in]
            n145 = property on="Command Selection" class="MCListbox (strict)"("ItemNames"=w253) -> ()  [unwired: 2 in, 2 out]
            n146 = property on="Command Params" class="Tbl (strict)"("Active Cell"=w263, "Cell BG Color"=w262, "Active Cell"=w261, "Cell BG Color"=w260) -> ()  [unwired: 2 in, 2 out]
            n147 = call <vilib>:"WPI_DashboardUpdate Command Params.vi"("Update"=w254, "NewVal"=w255, "Commands"=w253, "Param Tbl"=w252) -> ()  [unwired: 7 in, 1 out]
          }
        }
        n148 = call <vilib>:"Connextion Info.vi"() -> ("Connected"=→"NT Connection":bool)  [unwired: 10 in, 1 out]
      }
      event "Test Tree": Value Change {
        # "Show appropriate\ncontrols"
        n149 = event-data() -> ("CtlRef"=w269:refnum<vi>, "NewVal"=w267:string)  [unwired: 1 in]
        n150 = call <vilib>:"WPI_UtilitiesGetTreeIOName.vi"("NewVal"=w267, "TreeControl in"=w269) -> ("I/O Name"=w270:string)  [unwired: 9 in]
        n151 = case shown="\"Camera\"" w270 {
          selector: w270 -> [_ w277 _ w299 w308 _]
          tunnel: w267 -> [_ _ w296 w298 _ w315]
          tunnel: cluster{string[]}[] [{["640x480", "320x240", "160x120"]}, {["Auto", "Fixed indoor", "Fixed outdoor 1", "Fixed outdoor 2", "Fixed fluorescent 1", "Fixed fluorescent 2", "Hold current"]}, {["Auto", "Flicker-free 50 Hz", "Flicker-free 60 Hz", "Hold current"]}, {["None", "Prioritize frame rate", "Prioritize image quality"]}, {["Monochrome", "Color"]}] -> [_ _ _ _ _ w314]
          frame Default {
            w272 = FALSE ("Visible")
            w271 = FALSE ("Visible")
            n152 = property on="Motor" class="Clust (strict)"("Visible"=w271) -> ()  [unwired: 2 in, 2 out]
            n153 = property on="Test Ring" class="Ring (strict)"("Visible"=w271) -> ()  [unwired: 2 in, 2 out]
            n154 = property on="Rev/Fwd" class="Clust (strict)"("Visible"=w272) -> ()  [unwired: 2 in, 2 out]
            n155 = property on="On/Off" class="Bool (strict)"("Visible"=w272) -> ()  [unwired: 2 in, 2 out]
            n156 = property on="Test Slider" class="Slide (strict)"("Visible"=w272) -> ()  [unwired: 2 in, 2 out]
          }
          frame "Analog Out", "Motor", "PWM" {
            w278 = FALSE ("Visible")
            n157 = case shown="\"Analog Out\"" w277 {
              tunnel: [1.0 ("Value") -1.0 ("Value") 0.0 ("Value")] -> w276
              tunnel: [255.0 ("Value") 1.0 ("Value") 5.0 ("Value")] -> w275
              tunnel: [128.0 ("Value") 0.0 ("Value") 0.0 ("Value")] -> w274
              tunnel: [64.0 ("Value") 0.5 ("Value") 1.0 ("Value")] -> w273
              frame "PWM" {
              }
              frame "Motor", Default {
              }
              frame "Analog Out" {
              }
            }
            n158 = property on="Motor" class="Clust (strict)"("Visible"=TRUE) -> ()  [unwired: 2 in, 2 out]
            n159 = property on="Value" class="Slide (strict)"("Value"=w274, "Scale.Minimum"=w276, "Scale.Maximum"=w275, "Scale.Increment"=w273) -> ()  [unwired: 2 in, 2 out]
            n160 = property on="On/Off" class="Bool (strict)"("Visible"=w278) -> ()  [unwired: 2 in, 2 out]
            n161 = property on="Test Slider" class="Slide (strict)"("Visible"=w278) -> ()  [unwired: 2 in, 2 out]
            n162 = property on="Test Ring" class="Ring (strict)"("Visible"=w278) -> ()  [unwired: 2 in, 2 out]
            n163 = property on="Rev/Fwd" class="Clust (strict)"("Visible"=w278) -> ()  [unwired: 2 in, 2 out]
          }
          frame "Servo" {
            w294 = FALSE ("Visible")
            n164 = call <vilib>:"NT Read Number.vi"("Name"=w296) -> ("Numeric"=w295:dbl)  [unwired: 9 in, 1 out]
            n165 = property on="Test Slider" class="Slide (strict)"("Visible"=TRUE, "Scale.Maximum"=170.0 ("Scale.Range:Maximum")) -> ()  [unwired: 2 in, 2 out]
            n166 = local write "Test Slider"(w295) -> ()
            n167 = property on="Motor" class="Clust (strict)"("Visible"=w294) -> ()  [unwired: 2 in, 2 out]
            n168 = property on="Rev/Fwd" class="Clust (strict)"("Visible"=w294) -> ()  [unwired: 2 in, 2 out]
            n169 = property on="On/Off" class="Bool (strict)"("Visible"=w294) -> ()  [unwired: 2 in, 2 out]
            n170 = property on="Test Ring" class="Ring (strict)"("Visible"=w294) -> ()  [unwired: 2 in, 2 out]
          }
          frame "Relay", "Solenoid" {
            w297 = FALSE ("Visible")
            n171 = property on="Motor" class="Clust (strict)"("Visible"=w297) -> ()  [unwired: 2 in, 2 out]
            n172 = property on="Test Slider" class="Slide (strict)"("Visible"=w297) -> ()  [unwired: 2 in, 2 out]
            n173 = Search and Replace String(input string=w298, search string="/Value  **", replace string="/Direction") -> (result string=w304:string)  [unwired: 5 in, 3 out]
            n174 = property on="Test Ring" class="Ring (strict)"("Visible"=w297) -> ()  [unwired: 2 in, 2 out]
            n175 = call <vilib>:"NT Read String.vi"("Name"=w304) -> ("String"=w302:string)  [unwired: 9 in, 1 out]
            n176 = Equal?(x="Both directions", y=w302) -> (x = y?=w300:bool)
            n177 = Not(x=w300) -> (.not. x?=w301:bool)
            n178 = property on="Rev/Fwd" class="Clust (strict)"("Visible"=w300) -> ()  [unwired: 2 in, 2 out]
            n179 = property on="On/Off" class="Bool (strict)"("Visible"=w301, "Caption.Text"=w299) -> ()  [unwired: 2 in, 2 out]
          }
          frame "Compressor", "Digital Out" {
            w307 = FALSE ("Visible")
            # "Get direction and finish"
            n180 = property on="Motor" class="Clust (strict)"("Visible"=w307) -> ()  [unwired: 2 in, 2 out]
            n181 = property on="Test Slider" class="Slide (strict)"("Visible"=w307) -> ()  [unwired: 2 in, 2 out]
            n182 = property on="Test Ring" class="Ring (strict)"("Visible"=w307) -> ()  [unwired: 2 in, 2 out]
            n183 = property on="On/Off" class="Bool (strict)"("Visible"=TRUE, "Caption.Text"=w308) -> ()  [unwired: 2 in, 2 out]
            n184 = property on="Rev/Fwd" class="Clust (strict)"("Visible"=FALSE) -> ()  [unwired: 2 in, 2 out]
          }
          frame "Camera" {
            n185 = call <vilib>:"Get Last Path Segment.vi"("String in"=w315) -> ("String out"=w316:string)  [unwired: 10 in]
            n186 = property on="On/Off" class="Bool (strict)"("Visible"=FALSE) -> ()  [unwired: 2 in, 2 out]
            n187 = property on="Motor" class="Clust (strict)"("Visible"=FALSE) -> ()  [unwired: 2 in, 2 out]
            n188 = property on="Rev/Fwd" class="Clust (strict)"("Visible"=FALSE) -> ()  [unwired: 2 in, 2 out]
            n189 = case shown="\"White Balance  **\"" w316 {
              tunnel: w315 -> [w322 w331 w340 w349 w358 _ w364]
              tunnel: w314 -> [w320 w328 w337 w346 w355 _ _]
              frame "Size  **" {
                n190 = Index Array(array=w320) -> (element=w319:cluster{string[]})  [unwired: 1 in]
                n191 = call <vilib>:"NT Read String.vi"("Name"=w322) -> ("String"=w321:string)  [unwired: 9 in, 1 out]
                n192 = Unbundle(w319) -> (w317:string[])
                n193 = Match First String(2:w317, 3:w321) -> (0:w318:i32)  [unwired: 1 out]
                n194 = property on="Test Ring" class="Ring (strict)"("Value"=w318, "Strings []"=w317) -> ()  [unwired: 2 in, 2 out]
                n195 = property on="Test Ring" class="Ring (strict)"("Visible"=TRUE) -> ()  [unwired: 2 in, 2 out]
                n196 = property on="Test Slider" class="Slide (strict)"("Visible"=FALSE) -> ()  [unwired: 2 in, 2 out]
              }
              frame "White Balance  **" {
                n197 = Index Array(array=w328, index=1) -> (element=w329:cluster{string[]})
                n198 = call <vilib>:"NT Read String.vi"("Name"=w331) -> ("String"=w330:string)  [unwired: 9 in, 1 out]
                n199 = Unbundle(w329) -> (w326:string[])
                n200 = Match First String(2:w326, 3:w330) -> (0:w325:i32)  [unwired: 1 out]
                n201 = property on="Test Ring" class="Ring (strict)"("Value"=w325, "Strings []"=w326) -> ()  [unwired: 2 in, 2 out]
                n202 = property on="Test Ring" class="Ring (strict)"("Visible"=TRUE) -> ()  [unwired: 2 in, 2 out]
                n203 = property on="Test Slider" class="Slide (strict)"("Visible"=FALSE) -> ()  [unwired: 2 in, 2 out]
              }
              frame "Exposure  **" {
                n204 = Index Array(array=w337, index=2) -> (element=w338:cluster{string[]})
                n205 = call <vilib>:"NT Read String.vi"("Name"=w340) -> ("String"=w339:string)  [unwired: 9 in, 1 out]
                n206 = Unbundle(w338) -> (w334:string[])
                n207 = Match First String(2:w334, 3:w339) -> (0:w335:i32)  [unwired: 1 out]
                n208 = property on="Test Ring" class="Ring (strict)"("Value"=w335, "Strings []"=w334) -> ()  [unwired: 2 in, 2 out]
                n209 = property on="Test Ring" class="Ring (strict)"("Visible"=TRUE) -> ()  [unwired: 2 in, 2 out]
                n210 = property on="Test Slider" class="Slide (strict)"("Visible"=FALSE) -> ()  [unwired: 2 in, 2 out]
              }
              frame "Exposure Priority  **" {
                n211 = Index Array(array=w346, index=3) -> (element=w347:cluster{string[]})
                n212 = call <vilib>:"NT Read String.vi"("Name"=w349) -> ("String"=w348:string)  [unwired: 9 in, 1 out]
                n213 = Unbundle(w347) -> (w343:string[])
                n214 = Match First String(2:w343, 3:w348) -> (0:w344:i32)  [unwired: 1 out]
                n215 = property on="Test Ring" class="Ring (strict)"("Value"=w344, "Strings []"=w343) -> ()  [unwired: 2 in, 2 out]
                n216 = property on="Test Ring" class="Ring (strict)"("Visible"=TRUE) -> ()  [unwired: 2 in, 2 out]
                n217 = property on="Test Slider" class="Slide (strict)"("Visible"=FALSE) -> ()  [unwired: 2 in, 2 out]
              }
              frame "Color Enable  **" {
                n218 = Index Array(array=w355, index=4) -> (element=w356:cluster{string[]})
                n219 = call <vilib>:"NT Read String.vi"("Name"=w358) -> ("String"=w357:string)  [unwired: 9 in, 1 out]
                n220 = Unbundle(w356) -> (w352:string[])
                n221 = Match First String(2:w352, 3:w357) -> (0:w353:i32)  [unwired: 1 out]
                n222 = property on="Test Ring" class="Ring (strict)"("Value"=w353, "Strings []"=w352) -> ()  [unwired: 2 in, 2 out]
                n223 = property on="Test Ring" class="Ring (strict)"("Visible"=TRUE) -> ()  [unwired: 2 in, 2 out]
                n224 = property on="Test Slider" class="Slide (strict)"("Visible"=FALSE) -> ()  [unwired: 2 in, 2 out]
              }
              frame Default {
                n225 = property on="Test Ring" class="Ring (strict)"("Visible"=FALSE) -> ()  [unwired: 2 in, 2 out]
                n226 = property on="Test Slider" class="Slide (strict)"("Visible"=FALSE) -> ()  [unwired: 2 in, 2 out]
              }
              frame "Brightness  **", "Color Level  **", "Compression  **", "FPS  **", "Sharpness  **" {
                n227 = call <vilib>:"NT Read Number.vi"("Name"=w364) -> ("Numeric"=w363:dbl)  [unwired: 9 in, 1 out]
                n228 = local write "Test Slider"(w363) -> ()
                n229 = property on="Test Slider" class="Slide (strict)"("Visible"=TRUE, "Scale.Maximum"=100.0 ("Scale.Range:Maximum")) -> ()  [unwired: 2 in, 2 out]
                n230 = property on="Test Ring" class="Ring (strict)"("Visible"=FALSE) -> ()  [unwired: 2 in, 2 out]
              }
            }
          }
        }
        n231 = property on="Progress" class="Clust (strict)"("Visible"=FALSE) -> ()  [unwired: 2 in, 2 out]
      }
      event "Test Name": Mouse Enter {
        # "Populate the ring with the list of tests"
        n232 = event-data() -> ()  [unwired: 1 in, 1 out]
        n233 = call <vilib>:"NT Read String Array.vi"("Name"="TestMode/TestList") -> ("String Array"=w372:string[])  [unwired: 9 in, 1 out]
        n234 = Build Array (concatenate)("Select the test to run...", w372) -> (w371:string[])
        n235 = property on="Test Name" class="Ring (strict)"("Strings []"=w371) -> ()  [unwired: 2 in, 2 out]
      }
      event "Test Name": Value Change {
        w374 = FALSE ("Visible")
        # "Tell the robot the test name to run"
        n236 = event-data() -> ("NewVal"=w378:u16)  [unwired: 1 in]
        n237 = property on="Test Name" class="Ring (strict)"() -> ("Strings []"=w379:string[])  [unwired: 2 in, 2 out]
        n238 = local write "Progress"(T6 {"Test Progress"=0, "Test Progress Text"=""} ("Progress")) -> ()
        n239 = Index Array(array=w379, index=w378) -> (element=w377:string)
        n240 = call <vilib>:"NT Write String.vi"("String"=w377, "Name"="TestMode/TestName") -> ()  [unwired: 9 in, 1 out]
        n241 = property on="Progress" class="Clust (strict)"("Visible"=TRUE) -> ()  [unwired: 2 in, 2 out]
        n242 = property on="Motor" class="Clust (strict)"("Visible"=w374) -> ()  [unwired: 2 in, 2 out]
        n243 = property on="Test Slider" class="Slide (strict)"("Visible"=w374) -> ()  [unwired: 2 in, 2 out]
        n244 = property on="On/Off" class="Bool (strict)"("Visible"=w374) -> ()  [unwired: 2 in, 2 out]
        n245 = property on="Rev/Fwd" class="Clust (strict)"("Visible"=w374) -> ()  [unwired: 2 in, 2 out]
        n246 = property on="Test Ring" class="Ring (strict)"("Visible"=w374) -> ()  [unwired: 2 in, 2 out]
      }
      event "Select Auto": Mouse Enter {
        # "Populate the combo box with the list of autonomous options"
        n247 = event-data() -> ()  [unwired: 1 in, 1 out]
        n248 = call <vilib>:"NT Read String Array.vi"("Name"="Auto List") -> ("String Array"=w381:string[])  [unwired: 9 in, 1 out]
        n249 = property on="Select Auto" class="CmbBox"("Strings[]"=w381) -> ()  [unwired: 2 in, 2 out]
      }
      event "Select Auto": Value Change {
        # "User modified the Auto Selection. Write to NT variable so robot knows."
        n250 = event-data() -> ("NewVal"=w384:string)  [unwired: 1 in]
        n251 = call <vilib>:"NT Write String.vi"("String"=w384, "Name"="Auto Selector") -> ()  [unwired: 9 in, 1 out]
      }
      event "Command Selection": Value Change {
        # "Get the params and show in table"
        n252 = event-data() -> ("NewVal"=w390:i32)  [unwired: 1 in]
        n253 = property on="Command Selection" class="MCListbox (strict)"() -> ("ItemNames"=w388:string[][])  [unwired: 2 in, 2 out]
        n254 = call <vilib>:"WPI_DashboardUpdate Command Params.vi"("NewVal"=w390, "Commands"=w388, "Param Tbl"=w389) -> ()  [unwired: 8 in, 1 out]
      }
      event "Execute Command": Value Change {
        # "Started one, Unique ID holds\nresponse"
        n255 = event-data() -> ()  [unwired: 1 in, 1 out]
        n256 = property on="Command Selection" class="MCListbox (strict)"() -> ("ItemNames"=w401:string[][])  [unwired: 2 in, 2 out]
        n257 = Index Array(array=w401, index (row)="Command Selection", index (col)=0) -> (element=w399:string)
        n258 = call <vilib>:"Invoke Commands.vi"("Command Params"="Command Params", "Function Name"=w399) -> ("Params"=w395:u8, "Started"=w394:bool)  [unwired: 7 in, 1 out]
        n259 = Array Subset(array="Command Params", length (row)=w395) -> (w396:string[][])  [unwired: 3 in]
        n260 = Select(t="Executing" ("Cmd Status"), s=w394, f="" ("Cmd Status")) -> (s? t:f=→"Cmd Status":string)
      }
      event "Command Selection": Double Click {
        n261 = event-data() -> ("Row"=w409:i32)  [unwired: 1 in]
        n262 = property on="Command Selection" class="MCListbox (strict)"() -> ("ItemNames"=w412:string[][])  [unwired: 2 in, 2 out]
        n263 = local read "Command Params"() -> (w408:string[][])
        n264 = Index Array(array=w412, index (row)=w409, index (col)=0) -> (element=w410:string)
        n265 = call <vilib>:"Invoke Commands.vi"("Command Params"=w408, "Function Name"=w410) -> ("Params"=w407:u8, "Started"=w402:bool)  [unwired: 7 in, 1 out]
        n266 = Array Subset(array=w408, length (row)=w407) -> (w406:string[][])  [unwired: 3 in]
        n267 = Select(t="Executing" ("Cmd Status"), s=w402, f="" ("Cmd Status")) -> (s? t:f=w403:string)
        n268 = local write "Cmd Status"(w403) -> ()
      }
      event "CheckList": Double Click {
        # "Shift clears all"
        # "Update symbols on the listbox"
        n269 = event-data() -> ("PlatMods.Shift"=w414:bool, "Row"=w416:i32)  [unwired: 1 in]
        n270 = case shown="True" w414 {
          tunnel: w416 -> [w420 _]
          tunnel: 1 -> [w419 _]
          frame False {
            n271 = property on="CheckList" class="LstBox (strict)"() -> ("Item Symbols"=w418:i32[])  [unwired: 2 in, 2 out]
            n272 = Replace Array Subset(array=w418, new element=w419, index=w420) -> (w417:i32[])
            n273 = property on="CheckList" class="LstBox (strict)"("Item Symbols"=w417) -> ()  [unwired: 2 in, 2 out]
          }
          frame True {
            w421 = 0 ("Top Row")
            n274 = property on="CheckList" class="LstBox (strict)"() -> ("Number of Rows"=w423:u32)  [unwired: 2 in, 2 out]
            n275 = Initialize Array(0, w423) -> (w422:i32[])
            n276 = property on="CheckList" class="LstBox (strict)"("Top Row"=w421, "Value"=w421, "Item Symbols"=w422) -> ()  [unwired: 2 in, 2 out]
          }
        }
      }
      event "CheckList": Key Down {
        # "Update symbols on the listbox\nLeft and right keys check and uncheck"
        n277 = event-data() -> ("VKey"=w427:T23)  [unwired: 1 in]
        n278 = case shown="\"Left\", \"Right\"" w427 {
          selector: w427 -> [w432 _]
          tunnel: eventvkey."Left" ("VKey") -> [w430 _]
          frame "Left", "Right" {
            n279 = Equal?(x=w430, y=w432) -> (x = y?=w431:bool)
            n280 = Select(t=0, s=w431, f=1) -> (s? t:f=w433:i32)
            n281 = property on="CheckList" class="LstBox (strict)"() -> ("Item Symbols"=w436:i32[])  [unwired: 2 in, 2 out]
            n282 = Replace Array Subset(array=w436, new element=w433, index="CheckList") -> (w435:i32[])
            n283 = property on="CheckList" class="LstBox (strict)"("Item Symbols"=w435) -> ()  [unwired: 2 in, 2 out]
          }
          frame Default {
          }
        }
      }
      event "Motor.Enable": Value Change {
        # "When the test mode otor enable helper is set, update that\ntree row item's value"
        n284 = event-data() -> ("NewVal"=w442:bool)  [unwired: 1 in]
        n285 = Unbundle("Motor") -> ("Value"=w441:dbl)  [unwired: 1 out]
        n286 = Select(t=w441, s=w442, f=0.0) -> (s? t:f=w439:dbl)
        n287 = call <vilib>:"NT Write Number.vi"("Numeric"=w439, "Name"=w438) -> ()  [unwired: 9 in, 1 out]
      }
      event "Test Slider": Value Change {
        # "When the test mode slider helper is set, update that\ntree row item's value"
        n288 = event-data() -> ("NewVal"=w445:dbl)  [unwired: 1 in]
        n289 = call <vilib>:"NT Write Number.vi"("Numeric"=w445, "Name"=w446) -> ()  [unwired: 9 in, 1 out]
      }
      event "On/Off": Value Change {
        # "When the test mode on/off helper value is set, update that\ntree row item's value"
        n290 = event-data() -> ("NewVal"=w450:bool)  [unwired: 1 in]
        n291 = Boolean To (0,1)(Boolean=w450) -> (0, 1=w449:i16)
        n292 = call <vilib>:"NT Write Number.vi"("Numeric"=w449, "Name"=w448) -> ()  [unwired: 9 in, 1 out]
      }
      event "Rev/Fwd": Value Change {
        # "When the test mode helper value for relays is set, update that\ntree row item's value"
        n293 = event-data() -> ("NewVal.Forward"=w458:bool, "NewVal.Reverse"=w457:bool)  [unwired: 1 in]
        n294 = Boolean To (0,1)(Boolean=w458) -> (0, 1=w454:i16)
        n295 = Boolean To (0,1)(Boolean=w457) -> (0, 1=w456:i16)
        n296 = Negate(x=w456) -> (-x=w455:i16)
        n297 = Add(x=w454, y=w455) -> (x+y=w453:i16)
        n298 = call <vilib>:"NT Write Number.vi"("Numeric"=w453, "Name"=w452) -> ()  [unwired: 9 in, 1 out]
      }
      event "Test Ring": Value Change {
        # "When a test mode helper value is selected from the ring,\nset the tree item's variable to the string value"
        n299 = event-data() -> ("NewVal"=w462:u16)  [unwired: 1 in]
        n300 = property on="Test Ring" class="Ring (strict)"() -> ("Strings []"=w463:string[])  [unwired: 2 in, 2 out]
        n301 = Index Array(array=w463, index=w462) -> (element=w461:string)
        n302 = call <vilib>:"NT Write String.vi"("String"=w461, "Name"=w460) -> ()  [unwired: 9 in, 1 out]
      }
      event "Rec Mode": Value Change {
        # "Update globals for recording mode and path to read log from.\nClear when logging and let NetworkTables set path for vision to\nuse."
        n303 = event-data() -> ("NewVal"=w474:enum32{"Stop", "Record", "Playback"})  [unwired: 1 in]
        n304 = global write "WPI_DashboardLogging Global.vi" "Logging Filename"(path "") -> ()
        n305 = global write "WPI_DashboardLogging Global.vi" "Recording"(w474) -> ()
        n306 = case shown="\"Playback\"" w474 {
          tunnel: w473 -> [_ w476 w485]
          tunnel: [_ _ w484] -> w471
          tunnel: [_ _ w483] -> _
          tunnel: w469 -> [_ _ w481]
          tunnel: cluster{i32, i32} {-250, 170} -> [_ _ w480]
          tunnel: [_ _ T24 {"Image Size"=TRUE, "Image Type"=TRUE, "Pixel Value"=TRUE, "ROI Information"=TRUE, "Zoom Factor"=FALSE} ("Image Information Shown:All Elements")] -> w464
          tunnel: [_ _ TRUE ("Zoom Factor")] -> w465
          tunnel: w467 -> [_ _ w477]
          frame Default {
          }
          frame "Stop", "Record" {
            # "Place Window too"
            n307 = invoke class="VI" method="FP.Close"(reference=w476) -> (reference out=w475:refnum<vi>)  [unwired: 2 in, 2 out]
            n308 = invoke class="VI" method="Abort VI"(reference=w475) -> ()  [unwired: 2 in, 3 out]
          }
          frame "Playback" {
            n309 = call "Open Playback Panel.vi"("Offset"=w480, "DB VI Ref"=w481, "Playback in"=w485) -> ("Playback out"=w482:refnum<vi>)  [unwired: 8 in]
            n310 = register-events(w482, w477) -> (reference out=w484:refnum<event-registration>, error out=w483:errorcluster)  [unwired: 2 in]
          }
        }
        n311 = property on="Camera Image Right" class="ImageControl"("Image Information Shown"=w464, "Image Information Visible"=w465) -> ()  [unwired: 2 in, 2 out]
        n312 = property on="Camera Image" class="ImageControl"("Image Information Shown"=w464, "Image Information Visible"=w465) -> ()  [unwired: 2 in, 2 out]
        n313 = call <vilib>:"WPI_DashboardNT Log FieldName Cache.vi"("Operation"=enum16{"Lookup/Add", "Index", "Clear"}."Clear") -> ()  [unwired: 8 in, 3 out]
      }
      event Panel Close {
        w487 = enum32{"Stop", "Record", "Playback"}."Stop" ("Rec Mode")
        # "Playback window has been closed, abort"
        n314 = event-data() -> ()  [unwired: 1 in, 4 out]
        n315 = local write "Rec Mode"(w487) -> ()
        n316 = global write "WPI_DashboardLogging Global.vi" "Recording"(w487) -> ()
      }
      event Panel Close {
        # "Abort playback window and ourself"
        n317 = event-data() -> ()  [unwired: 1 in, 4 out]
        n318 = invoke class="VI" method="FP.Close"(reference=w491) -> (reference out=w490:refnum<vi>)  [unwired: 2 in, 2 out]
        n319 = invoke class="VI" method="Abort VI"(reference=w490) -> (error out=w489:errorcluster)  [unwired: 2 in, 2 out]
        n320 = invoke class="VI" method="Abort VI"(error in=w489) -> ()  [unwired: 2 in, 3 out]
      }
      event User Event {
        n321 = event-data() -> ("IDs"=w498:cluster{"RPC field ID":u16, "Unique ID":u16}, "String"=w497:string)  [unwired: 1 in]
        n322 = Bundle("IDs"=w498, "String"=w497) -> (w496:T10)  [unwired: 1 in]
        n323 = call <vilib>:"Retrieve RPC Response.vi"("RPC Response"=w496) -> ("Output"=w494:string[][])  [unwired: 10 in]
        n324 = Build Array (concatenate)(w492, w494) -> (w493:string[][])
        n325 = local write "Command Params"(w493) -> ()
        n326 = local write "Cmd Status"("" ("Cmd Status")) -> ()
      }
      event "Tree": Double Click {
        n327 = event-data() -> ("PlatMods"=w504:T27, "Tag"=w501:string)  [unwired: 1 in]
        n328 = Unbundle(w504) -> ("Shift"=w503:bool)  [unwired: 4 out]
        n329 = String Subset(string=w501, length (rest)=1 ("length (rest)")) -> (substring=w500:string)  [unwired: 1 in]
        n330 = Not(x=w503) -> (.not. x?=w502:bool)
        n331 = case shown="\"/\"" w500 {
          tunnel: w501 -> [_ w507]
          tunnel: w502 -> [_ w506]
          frame Default {
          }
          frame "/" {
            n332 = call <vilib>:"NT Update Persistence.vi"("Persistence"=w506, "Name"=w507) -> ()  [unwired: 9 in, 1 out]
          }
        }
      }
    }
  }
  n333 = while {
    tunnel: w65 -> [w509]
    i -> [w512]
    stop <- FALSE stop-if-true
    n334 = Wait (ms)(milliseconds to wait=u32 100) -> ()  [unwired: 1 out]
    n335 = case shown="\"Playback\"" "Rec Mode" {
      tunnel: w512 -> [_ _ w527]
      tunnel: [u32 2829099 ("Base Color") u32 11141120 ("Target Color") w516] -> w508
      frame "Stop", Default {
        # "Reset the color, extra updates don't cost much"
      }
      frame "Record" {
      }
      frame "Playback" {
        # "Playback"
        n336 = Quotient & Remainder(x=w527, y=u32 50 ("milliseconds to wait")) -> (x-y*floor(x/y)=w523:u32)  [unwired: 1 out]
        n337 = Divide(x=w523, y=u32 50 ("milliseconds to wait")) -> (x/y=w520:dbl)
        n338 = Multiply(x=6.283185307179586, y=w520) -> (x*y=w525:dbl)
        n339 = Sine(x=w525) -> (sin(x)=w524:dbl)
        n340 = Absolute Value(x=w524) -> (abs(x)=w517:dbl)
        n341 = call "Interpolate RGB Color.vi"("Proportion"=w517, "Target Color"=u32 30976, "Base Color"=u32 2829099) -> ("Result Color"=w516:u32)  [unwired: 8 in]
      }
    }
    n342 = property class="Pane"(reference=w509, "PaneColor"=w508) -> ()  [unwired: 1 in, 2 out]
  }
  n343 = local write "Dashboard Tab"(T2."Drive" ("Dashboard Tab")) -> ()
  n344 = property on="On/Off" class="Bool (strict)"("Visible"=w36) -> ()  [unwired: 2 in, 2 out]
  n345 = property on="Motor" class="Clust (strict)"("Visible"=w36) -> ()  [unwired: 2 in, 2 out]
  n346 = property on="Progress" class="Clust (strict)"("Visible"=w36) -> ()  [unwired: 2 in, 2 out]
  n347 = property on="Test Ring" class="Ring (strict)"("Visible"=w36) -> ()  [unwired: 2 in, 2 out]
  n348 = property on="Rev/Fwd" class="Clust (strict)"("Visible"=w36) -> ()  [unwired: 2 in, 2 out]
  n349 = local write "Command Selection"(u16 0 ("milliseconds to wait")) -> ()
  n350 = while {
    tunnel: u16 1741 ("timeout ms (25000)") -> [w529]
    stop <- FALSE stop-if-true
    n351 = TCP Create Listener(10:w529) -> (0:w528:errorcluster, 3:w530:refnum<k5>)  [unwired: 4 in, 1 out]
    n352 = case shown="No Error" w528 {
      selector: w528 -> [w532 _]
      tunnel: w530 -> [w533 _]
      frame No Error {
        n353 = while {
          tunnel: w533 -> [w536]
          tunnel: w532 -> [w535]
          stop <- FALSE stop-if-true
          n354 = TCP Wait On Listener(8:w535, 11:w536) -> (0:w537:errorcluster, 4:w538:refnum<k5>)  [unwired: 2 in, 3 out]
          n355 = local write "TCP"(w538) -> ()
          n356 = case shown="No Error" w537 {
            frame No Error {
            }
            frame Error {
              n357 = Wait (ms)(milliseconds to wait=u32 1000) -> ()  [unwired: 1 out]
            }
          }
        }
      }
      frame Error {
        n358 = Wait (ms)(milliseconds to wait=u32 1000) -> ()  [unwired: 1 out]
      }
    }
  }
  n359 = local write "Command Params"(string[][] [] ("Command Params")) -> ()
  n360 = global write "WPI_DashboardLogging Global.vi" "Recording"(w59) -> ()
  n361 = local write "Rec Mode"(w59) -> ()
  n362 = call <vilib>:"NT Write String.vi"("String"="Select Auto", "Name"="Auto Selector") -> ()  [unwired: 9 in, 1 out]
